vi "NXTSumoEyes-Direct.vi"() -> ()   [LabVIEW 2009]
uses:
  <vilib>/NXT/Subs/LVHSConnector.ctl
  <vilib>/NXT/Block Support/NXT_InputPort.ctl
panel:
  in  "Select Range":u16(ring)=6 items=["short"=5, "long"=6]
  in  "?":bool=TRUE
  out "Right":bool
  out "Left":bool
  in  "Input Port":T1 items=["Port 1", "Port 2", "Port 3", "Port 4"]
  in  "NXT":T2={"error"={"status"=FALSE, "code"=0, "source"=""}, "address"="", "NXT #"=-1, "Show Error"=TRUE}
  out "NXT dup":T2={"error"={"status"=FALSE, "code"=0, "source"=""}, "address"="", "NXT #"=-1, "Show Error"=TRUE}
  # "mindsensors.com\nCopyright (c) 2009 by mindsensors.com\nEmail: info (<at>) mindsensors (<dot>) com\n\nThis program is free software. You can redistribute it and/or modify\nit under the terms of the GNU General Public License as published by\nthe Free Software Foundation; version 3 of the License.\nRead the license at: http://www.gnu.org/licenses/gpl.txt"
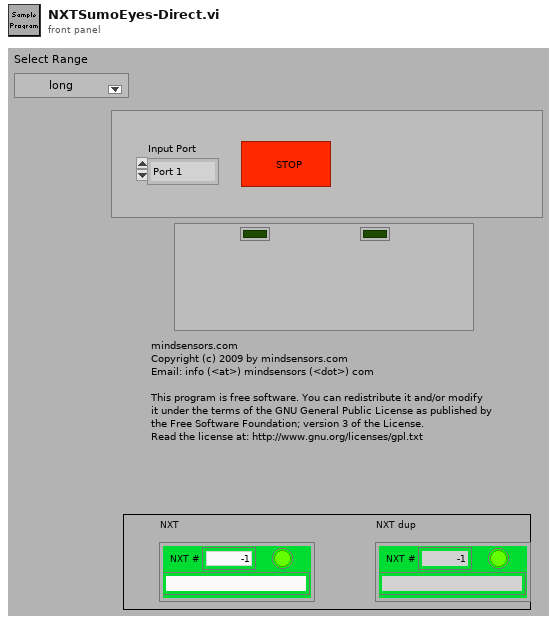
[diagram p1: front panel]
types:
  T1 = typedef "NXT_InputPort.ctl" = u8
  T2 = typedef "LVHSConnector.ctl" = cluster{"error":errorcluster, "address":string, "NXT #":i32, "Show Error":bool}
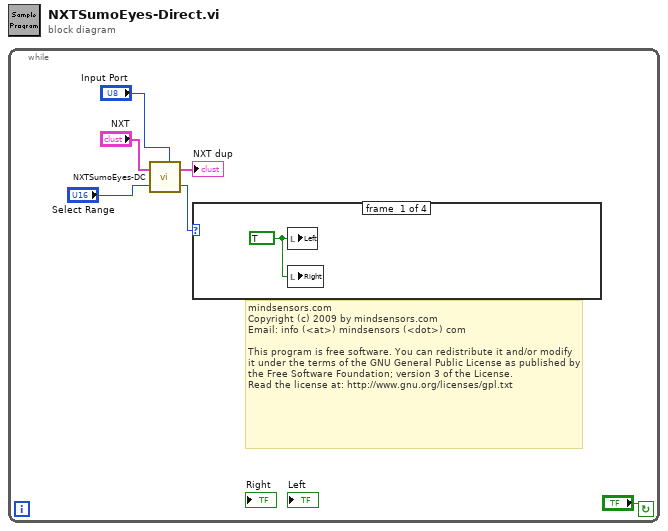
[diagram p0: block diagram]
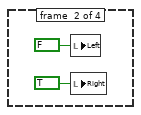
[diagram p2: hidden frame]
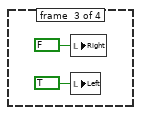
[diagram p3: hidden frame]
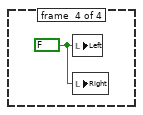
[diagram p4: hidden frame]
diagram:
  n1 = while {
    stop <- "?" continue-if-true
    # "mindsensors.com\nCopyright (c) 2009 by mindsensors.com\nEmail: info (<at>) mindsensors (<dot>) com\n\nThis program is free software. You can redistribute it and/or modify\nit under the terms of the GNU General Public License as published by\nthe Free Software Foundation; version 3 of the License.\nRead the license at: http://www.gnu.org/licenses/gpl.txt"
    n2 = call "NXTSumoEyes-DC.vi"("Select Range"="Select Range", "NXT"="NXT", "Input Port"="Input Port") -> ("What Zone?"=w2:u8, "NXT dup"=→"NXT dup":T2)  [unwired: 1 in, 1 out]
    n3 = case shown="1" w2 {
      frame #0 {
        w7 = TRUE
        n4 = local write "Left"(w7) -> ()
        n5 = local write "Right"(w7) -> ()
      }
      frame #1 {
        n6 = local write "Left"(FALSE ("Left")) -> ()
        n7 = local write "Right"(TRUE ("Right")) -> ()
      }
      frame #2 {
        n8 = local write "Right"(FALSE ("Right")) -> ()
        n9 = local write "Left"(TRUE ("Left")) -> ()
      }
      frame #3 {
        w12 = FALSE ("Left")
        n10 = local write "Left"(w12) -> ()
        n11 = local write "Right"(w12) -> ()
      }
    }
  }
